vi "MGCC_BlkStart_main.vi"() -> ()   [LabVIEW 2016]
uses:
  Sub-VIs/MGCC_BlkStart_Globals.vi
  Communication/Global communication output.vi
  Communication/Global communication.vi
  Model Management/Global_MdlMgmt.vi
  <vilib>/imath/engines/lvmath2/RunTimeEngine/BuiltInFunctions/sets_unique/NIMS_sets_unique(GM).vi
  <instcachedir>/0/NIMS_sets_unique(GM)_A55EFC7C1FC44AA39E21562D64C6E0C8.lvgen/NIMS_sets_unique(GM)_A55EFC7C1FC44AA39E21562D64C6E0C8_002.vi
  <vilib>/imathl/engines/lvmath/Functions/Error Handling/Create Error.vi
  <vilib>/imath/engines/lvmath2/RunTimeEngine/VariableToken/Support/NIMS_Matrix Boolean Index to I32 Index.vi
  <vilib>/imath/engines/lvmath2/RunTimeEngine/IndexRead/NIMS M(V).vi
  <instcachedir>/0/NIMS M(V)_948FAC22C1C943948B75DA6190348614.lvgen/NIMS M(V)_948FAC22C1C943948B75DA6190348614_005.vi
  <vilib>/imath/engines/lvmath2/RunTimeEngine/BuiltInFunctions/size/NIMS_I32=size(GM,I32).vi
  <instcachedir>/0/NIMS_I32=size(GM,I32)_122058B1B3294FAEA5DC209B92B394E4.lvgen/NIMS_I32=size(GM,I32)_122058B1B3294FAEA5DC209B92B394E4_004.vi
  <vilib>/imath/engines/lvmath2/RunTimeEngine/BuiltInFunctions/zeros/NIMS_M=zeros(I32,I32).vi
  <vilib>/imath/engines/lvmath2/RunTimeEngine/ErrorHandling/NIMS_Create Error From Enums.vi
  <vilib>/imath/engines/lvmath2/RunTimeEngine/IndexReplace/NIMS M($,S)=M.vi
  <instcachedir>/0/NIMS M($,S)=M_4ED09617E62F4BDFBC079C86D2836811.lvgen/NIMS M($,S)=M_4ED09617E62F4BDFBC079C86D2836811_000.vi
  <vilib>/imath/engines/lvmath2/RunTimeEngine/RangeToken/NIMS_Range_R2 - Integer.vi
  <instcachedir>/0/NIMS_Range_R2 - Integer_89B873E74E6E489885E44F751DD9C6BF.lvgen/NIMS_Range_R2 - Integer_89B873E74E6E489885E44F751DD9C6BF_000.vi
  <vilib>/imath/engines/lvmath2/RunTimeEngine/CommandStatement/MC_CommandStatement_break.vi
  <vilib>/imath/engines/lvmath2/RunTimeEngine/IndexRead/NIMS M($,S).vi
  <instcachedir>/0/NIMS M($,S)_3E5749BBB62E49528D4765A77F1F6D98.lvgen/NIMS M($,S)_3E5749BBB62E49528D4765A77F1F6D98_000.vi
  <vilib>/imath/engines/lvmath2/RunTimeEngine/IndexRead/NIMS M(S,S).vi
  <instcachedir>/0/NIMS M(S,S)_AC51E74150A542F7991B9634C66F3096.lvgen/NIMS M(S,S)_AC51E74150A542F7991B9634C66F3096_000.vi
  <vilib>/imath/engines/lvmath2/RunTimeEngine/BitwiseOperatorToken/NIMS_Bitwise_Operator_Or.vi
  <instcachedir>/0/NIMS_Bitwise_Operator_Or_51E58CBCE6004B7AAA420A8AC17D98D6.lvgen/NIMS_Bitwise_Operator_Or_51E58CBCE6004B7AAA420A8AC17D98D6_001.vi
  <vilib>/imath/engines/lvmath2/RunTimeEngine/VariableToken/Support/NIMS_Vector Boolean Index to I32 Index.vi
  <vilib>/imath/engines/lvmath2/RunTimeEngine/IndexRead/NIMS M(V,S).vi
  <instcachedir>/0/NIMS M(V,S)_4A7282EC9BD94252BB5D44AC841A97D6.lvgen/NIMS M(V,S)_4A7282EC9BD94252BB5D44AC841A97D6_000.vi
  <vilib>/imath/engines/lvmath2/RunTimeEngine/IndexReplace/NIMS M(S,S)=V.vi
  <instcachedir>/0/NIMS M(S,S)=V_EB62F88436AB4BC9BC6D9B91CABDA9F1.lvgen/NIMS M(S,S)=V_EB62F88436AB4BC9BC6D9B91CABDA9F1_000.vi
  <vilib>/imath/engines/lvmath2/RunTimeEngine/BuiltInFunctions/findnz/NIMS_[3o]_findnz(GM).vi
  <instcachedir>/0/NIMS_[3o]_findnz(GM)_99A5867F30DB48758370F82C3149E97C.lvgen/NIMS_[3o]_findnz(GM)_99A5867F30DB48758370F82C3149E97C_003.vi
  <vilib>/imath/engines/lvmath2/RunTimeEngine/IndexRead/NIMS M(M,M).vi
  <instcachedir>/0/NIMS M(M,M)_43A52FFC48884BCB815E619CBD2E8DAE.lvgen/NIMS M(M,M)_43A52FFC48884BCB815E619CBD2E8DAE_004.vi
  <vilib>/imath/engines/lvmath2/RunTimeEngine/IndexReplace/NIMS M(S,S)=M.vi
  <instcachedir>/0/NIMS M(S,S)=M_920697704EC84E059D04F7603C52D16B.lvgen/NIMS M(S,S)=M_920697704EC84E059D04F7603C52D16B_000.vi
  <vilib>/imath/engines/lvmath2/RunTimeEngine/NodeEndStatement/NIMS_NodeEndStatement_Output.vi
  <instcachedir>/0/NIMS_NodeEndStatement_Output_53EC0D466D134D7ABD903AC30B43404B.lvgen/NIMS_NodeEndStatement_Output_53EC0D466D134D7ABD903AC30B43404B_002.vi
  <vilib>/imath/engines/lvmath2/RunTimeEngine/ErrorHandling/NIMS_Finalize Error.vi
  <vilib>/imath/engines/lvmath2/RunTimeEngine/IndexRead/NIMS V(V).vi
  <instcachedir>/0/NIMS V(V)_298D9CB7BFEB42B8BC8D9C3C28AE8C70.lvgen/NIMS V(V)_298D9CB7BFEB42B8BC8D9C3C28AE8C70_000.vi
  <vilib>/imath/engines/lvmath2/RunTimeEngine/BuiltInFunctions/is_membermx/NIMS_is_membermx(GV,GM).vi
  <instcachedir>/0/NIMS_is_membermx(GV,GM)_15846B44F49A470EB5DEBB7BCD07BEEA.lvgen/NIMS_is_membermx(GV,GM)_15846B44F49A470EB5DEBB7BCD07BEEA_000.vi
  <vilib>/imath/engines/lvmath2/RunTimeEngine/IndexRead/NIMS M(V,$).vi
  <instcachedir>/0/NIMS M(V,$)_21A5155762F74C04AE4EA67BEE0D3EF5.lvgen/NIMS M(V,$)_21A5155762F74C04AE4EA67BEE0D3EF5_004.vi
  <vilib>/imath/engines/lvmath2/RunTimeEngine/BuiltInFunctions/prod/NIMS_prod(GV).vi
  <instcachedir>/0/NIMS_prod(GV)_1D7C69903E9744BFBC8310E18FF565A3.lvgen/NIMS_prod(GV)_1D7C69903E9744BFBC8310E18FF565A3_000.vi
  <vilib>/imath/engines/lvmath2/RunTimeEngine/IndexRead/NIMS V(S).vi
  <instcachedir>/0/NIMS V(S)_0488751826AF41519A22953C041130DC.lvgen/NIMS V(S)_0488751826AF41519A22953C041130DC_000.vi
  <instcachedir>/0/NIMS V(S)_0488751826AF41519A22953C041130DC.lvgen/NIMS V(S)_0488751826AF41519A22953C041130DC_003.vi
  <vilib>/imath/engines/lvmath2/RunTimeEngine/IndexReplace/NIMS V(S)=S.vi
  <instcachedir>/0/NIMS V(S)=S_57E16554CB8B4B90AAB163894F717546.lvgen/NIMS V(S)=S_57E16554CB8B4B90AAB163894F717546_004.vi
  <vilib>/imath/engines/lvmath2/RunTimeEngine/BuiltInFunctions/findnz/NIMS_[1o]_findnz(GColV).vi
  <instcachedir>/0/NIMS_[1o]_findnz(GColV)_8556557C9365446B906472366DD9B2D8.lvgen/NIMS_[1o]_findnz(GColV)_8556557C9365446B906472366DD9B2D8_000.vi
  <vilib>/imath/engines/lvmath2/RunTimeEngine/IndexReplace/NIMS M(S,V)=S.vi
  <instcachedir>/0/NIMS M(S,V)=S_8B14C5B5036146CBA8049B2A1E37AE34.lvgen/NIMS M(S,V)=S_8B14C5B5036146CBA8049B2A1E37AE34_000.vi
  <instcachedir>/0/NIMS_NodeEndStatement_Output_53EC0D466D134D7ABD903AC30B43404B.lvgen/NIMS_NodeEndStatement_Output_53EC0D466D134D7ABD903AC30B43404B_015.vi
  <instcachedir>/0/NIMS_NodeEndStatement_Output_53EC0D466D134D7ABD903AC30B43404B.lvgen/NIMS_NodeEndStatement_Output_53EC0D466D134D7ABD903AC30B43404B_013.vi
  Finite State Machine/Sub-VIs/MGCC_FntStaMach_gobal.vi
panel:
  out "PVon":bool
  out "GENon":bool
  out "BESSon":bool
  in  "error in":errorcluster
  out "error out":errorcluster
  out "LCStatus":i32[][](array[numeric])
  out "SourceStatus":dbl[][](array[numeric])
  out "SourceNodes":dbl[][](array[numeric])
  out "VoltWarning":bool
  out "FreqWarning":bool
  out "Limits":dbl[](array[numeric])=[59.9, 60.1, 0.9, 1.1]
  out "BlackStart":bool[](array[boolean])=[TRUE, TRUE]
  out "LC":dbl[][](array[numeric])=[[10.0, 1.0], [11.0, 0.0], [12.0, 1.0]]
  out "ListofCrit":dbl[](array[numeric])=[10.0]
  out "MG_topology":dbl[][](array[numeric])=[[3.0, 2.0, 1.0, 0.0, 1.0], [3.0, 4.0, 1.0, 0.0, 2.0], [7.0, 3.0, 1.0, 0.0, 3.0], [4.0, 5.0, 1.0, 0.0, 4.0], [7.0, 8.0, 1.0, 0.0, 5.0], [9.0, 7.0, 1.0, 0.0, 6.0], [10.0, 9.0, 1.0, 0.0, 7.0], [10.0, 11.0, 1.0, 0.0, 8.0], [10.0, 12.0, 4.0, 1.0, 100.0], [10.0, 13.0, 2.0, 1.0, 100.0]]
  # "Copyright <2020> <The University of Tennessee at Knoxville and the University of Tennessee Research Foundation>\n\nRedistribution and use in source and binary forms, with or without modification, are permitted provided that the following conditions are met:\n\n1. Redistributions of source code must retain the above copyright notice, this list of conditions and the following disclaimer.\n\n2. Redistributions in binary form must reproduce the above copyright notice, this list of conditions and the following disclaimer in the documentation and/or other materials provided with the distribution.\n\n3. Neither the name of the copyright holder nor the names of its contributors may be used to endorse or promote products derived from this software without specific prior written permission.\n\nTHIS SOFTWARE IS PROVIDED BY THE COPYRIGHT HOLDERS AND CONTRIBUTORS \"AS IS\" AND ANY EXPRESS OR IMPLIED WARRANTIES, INCLUDING, BUT NOT LIMITED TO, THE IMPLIED WARRANTIES OF MERCHANTABILITY AND FITNESS FOR A PARTICULAR PURPOSE ARE DISCLAIMED. IN NO EVENT SHALL THE COPYRIGHT HOLDER OR CONTRIBUTORS BE LIABLE FOR ANY DIRECT, INDIRECT, INCIDENTAL, SPECIAL, EXEMPLARY, OR CONSEQUENTIAL DAMAGES (INCLUDING, BUT NOT LIMITED TO, PROCUREMENT OF SUBSTITUTE GOODS OR SERVICES; LOSS OF USE, DATA, OR PROFITS; OR BUSINESS INTERRUPTION) HOWEVER CAUSED AND ON ANY THEORY OF LIABILITY, WHETHER IN CONTRACT, STRICT LIABILITY, OR TORT (INCLUDING NEGLIGENCE OR OTHERWISE) ARISING IN ANY WAY OUT OF THE USE OF THIS SOFTWARE, EVEN IF ADVISED OF THE POSSIBILITY OF SUCH DAMAGE."
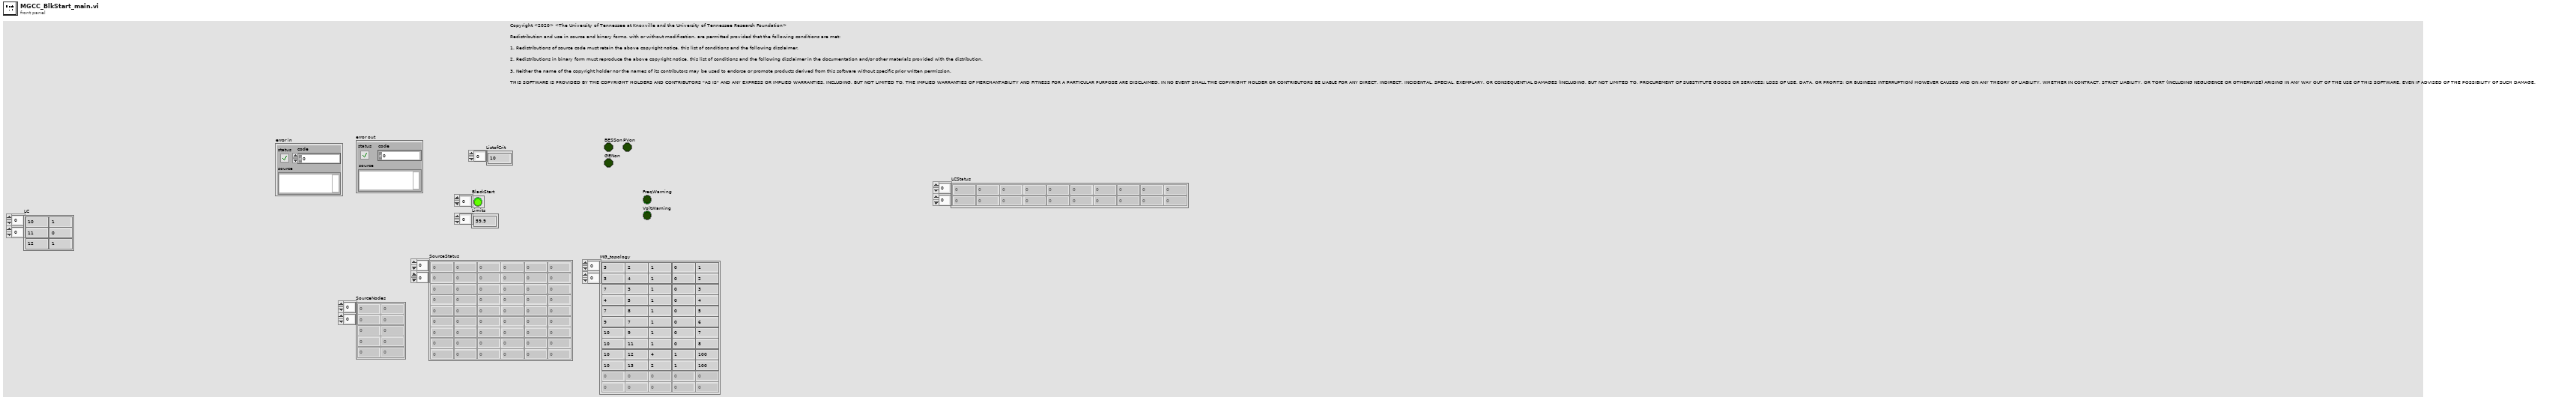
[diagram p1: front panel]
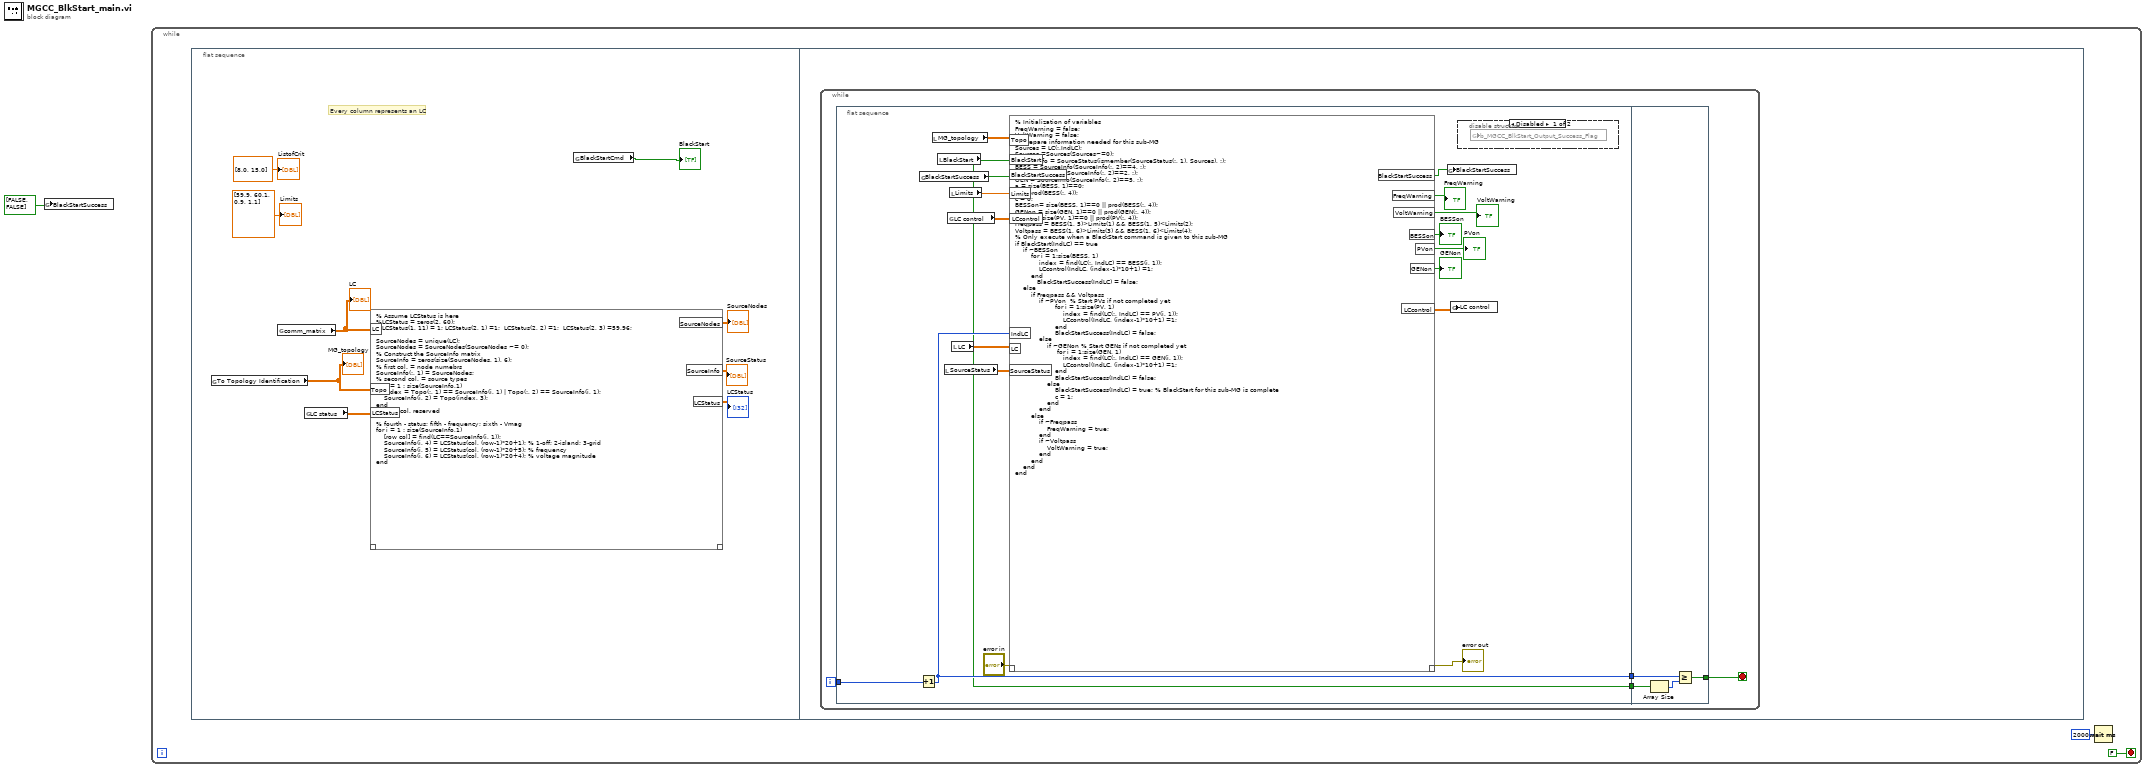
[diagram p0: block diagram]
diagram:
  n1 = global write "MGCC_BlkStart_Globals.vi" "BlackStartSuccess"(bool[] [FALSE, FALSE]) -> ()
  n2 = while {
    stop <- FALSE stop-if-true
    n3 = flat-sequence {
      frame #0 {
        # "Every column represents an LC"
        n4 = global read "Global_MdlMgmt.vi" "To Topology Identification"() -> (w5:dbl[][])
        "MG_topology" <- w5
        n5 = global read "Global communication output.vi" "comm_matrix"() -> (w8:dbl[][])
        "LC" <- w8
        n6 = global read "Global communication.vi" "LC status"() -> (w6:dbl[][])
        n7 = mathscript code="% Assume LCStatus is here\n%LCStatus = zeros(2, 60);\n%LCStatus(1, 11) = 1; LCStatus(2, 1) =1;  LCStatus(2, 2) =1;  LCStatus(2, 3) =59.96;\n\nSourceNodes = unique(LC);\nSourceNodes = SourceNodes(SourceNodes ~= 0);\n% Construct the SourceInfo matrix\nSourceInfo = zeros(size(SourceNodes, 1), 6);\n% first col. = node numebrs\nSourceInfo(:, 1) = SourceNodes;\n% second col. = source types\nfor i = 1 : size(SourceInfo,1)\n    index = Topo(:, 1) == SourceInfo(i, 1) | Topo(:, 2) == SourceInfo(i, 1);\n    SourceInfo(i, 2) = Topo(index, 3);\nend\n% third col. reserved\n\n% fourth - status; fifth - frequency; sixth - Vmag\nfor i = 1 : size(SourceInfo,1)\n    [row col] = find(LC==SourceInfo(i, 1));\n    SourceInfo(i, 4) = LCStatus(col, (row-1)*20+1); % 1-off; 2-island; 3-grid\n    SourceInfo(i, 5) = LCStatus(col, (row-1)*20+5); % frequency\n    SourceInfo(i, 6) = LCStatus(col, (row-1)*20+4); % voltage magnitude\nend"("LC"=w8, "Topo"=w5, "LCStatus"=w6) -> ("SourceNodes"=→"SourceNodes":dbl[][], "SourceInfo"=→"SourceStatus":dbl[][], "LCStatus"=→"LCStatus":dbl[][])  [unwired: 1 in, 1 out]
        n8 = global read "MGCC_BlkStart_Globals.vi" "BlackStartCmd"() -> (→"BlackStart":bool[])
        "ListofCrit" <- dbl[] [8.0, 15.0] ("ListofCrit")
        "Limits" <- dbl[] [59.9, 60.1, 0.9, 1.1]
      }
      frame #1 {
        n9 = while {
          i -> [w417]
          stop <- w414 stop-if-true
          n10 = flat-sequence {
            tunnel: w417 -> [w432]
            tunnel: [w428] -> w416
            tunnel: [w426] -> w415
            tunnel: w416 -> [w1605]
            tunnel: w415 -> [w1603]
            tunnel: [w1602] -> w414
            frame #0 {
              n11 = global read "MGCC_BlkStart_Globals.vi" "BlackStartSuccess"() -> (w420:bool[])
              n12 = Increment(x=w432) -> (x+1=w428:i32)
              n13 = local read "MG_topology"() -> (w435:dbl[][])
              n14 = local read "BlackStart"() -> (w426:bool[])
              n15 = local read "SourceStatus"() -> (w434:dbl[][])
              n16 = global read "Global communication.vi" "LC control"() -> (w427:dbl[][])
              n17 = local read "Limits"() -> (w431:dbl[])
              n18 = local read "LC"() -> (w433:dbl[][])
              n19 = mathscript code="% Initialization of variables\nFreqWarning = false;\nVoltWarning = false;\n% Prepare information needed for this sub-MG\nSources = LC(:,IndLC);\nSources =Sources(Sources~=0);\nSourceInfo = SourceStatus(ismember(SourceStatus(:, 1), Sources), :);\nBESS = SourceInfo(SourceInfo(:, 2)==4, :);\nPV = SourceInfo(SourceInfo(:, 2)==2, :);\nGEN = SourceInfo(SourceInfo(:, 2)==5, :);\na = size(BESS, 1)==0;\nb = prod(BESS(:, 4));\nc = 0;\nBESSon= size(BESS, 1)==0 || prod(BESS(:, 4));\nGENon = size(GEN, 1)==0 || prod(GEN(:, 4));\nPVon =  size(PV, 1)==0 || prod(PV(:, 4));\nFreqpass = BESS(1, 5)>Limits(1) && BESS(1, 5)<Limits(2);\nVoltpass = BESS(1, 6)>Limits(3) && BESS(1, 6)<Limits(4);\n% Only execute when a BlackStart command is given to this sub-MG\nif BlackStart(IndLC) == true\n    if ~BESSon\n        for i = 1:size(BESS, 1)\n            index = find(LC(:, IndLC) == BESS(i, 1));\n            LCcontrol(IndLC, (index-1)*10+1) =1;\n        end\n           BlackStartSuccess(IndLC) = false;\n    else\n        if Freqpass && Voltpass\n            if ~PVon  % Start PVs if not completed yet\n                    for i = 1:size(PV, 1)\n                        index = find(LC(:, IndLC) == PV(i, 1));\n                        LCcontrol(IndLC, (index-1)*10+1) =1;\n                    end\n                    BlackStartSuccess(IndLC) = false;\n            else\n                if ~GENon % Start GENs if not completed yet\n                     for i = 1:size(GEN, 1)\n                        index = find(LC(:, IndLC) == GEN(i, 1));\n                        LCcontrol(IndLC, (index-1)*10+1) =1;\n                    end\n                    BlackStartSuccess(IndLC) = false;\n                else\n                    BlackStartSuccess(IndLC) = true; % BlackStart for this sub-MG is complete\n                    c = 1;\n                end\n            end\n        else\n            if ~Freqpass\n                FreqWarning = true;\n            end\n            if ~Voltpass\n                VoltWarning = true;\n            end\n        end\n    end\nend"("??"="error in", "Topo"=w435, "BlackStart"=w426, "SourceStatus"=w434, "LC"=w433, "IndLC"=w428, "Limits"=w431, "BlackStartSuccess"=w420, "LCcontrol"=w427) -> ("??"=→"error out":errorcluster, "BlackStartSuccess"=w419:bool[], "FreqWarning"=→"FreqWarning":bool, "VoltWarning"=→"VoltWarning":bool, "BESSon"=→"BESSon":bool, "GENon"=→"GENon":bool, "PVon"=→"PVon":bool, "LCcontrol"=w418:dbl[][])
              n20 = global write "MGCC_BlkStart_Globals.vi" "BlackStartSuccess"(w419) -> ()
              n21 = global write "Global communication.vi" "LC control"(w418) -> ()
              n22 = disable-structure shown="Disabled" {
                frame Disabled {
                  n23 = global read "MGCC_FntStaMach_gobal.vi" "b_MGCC_BlkStart_Output_Success_Flag"() -> ()  [unwired: 1 in]
                }
                frame Enabled {
                }
              }
            }
            frame #1 {
              n24 = Array Size(array=w1603) -> (size(s)=w1604:i32)
              n25 = Greater Or Equal?(x=w1605, y=w1604) -> (x >= y?=w1602:bool)
            }
          }
        }
      }
    }
    n26 = Wait (ms)(milliseconds to wait=u32 2000) -> ()  [unwired: 1 out]
  }
